vi "Set Tx UDP Properties.vi"(8 "error in":errorcluster, 10 "session_tx_generic":cluster{"portId":u32, "VL":u32}, 11 "custom device ref in":T1 format="%.0x") -> (0 "error out":errorcluster, 3 "custom device ref out":T1 format="%.0x")   [LabVIEW 2020, in "AIM ARINC 664 Scripting.lvlib"]
uses:
  <vilib>/NI VeriStand/Custom Device API/Custom Device Item Ref.ctl
  Constants.vi
  <vilib>/NI VeriStand/Custom Device API/Set Item Property (U32).vi
  AIM ARINC 664 Scripting.lvlib
  <vilib>/NI VeriStand/Custom Device API/Custom Device API.lvlib
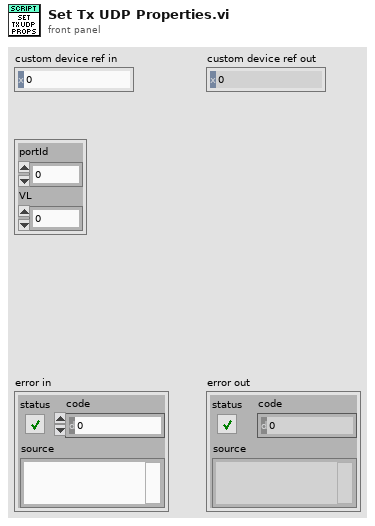
[diagram p1: front panel]
types:
  T1 = typedef "Custom Device API.lvlib/Custom Device Item Ref.ctl" = u64
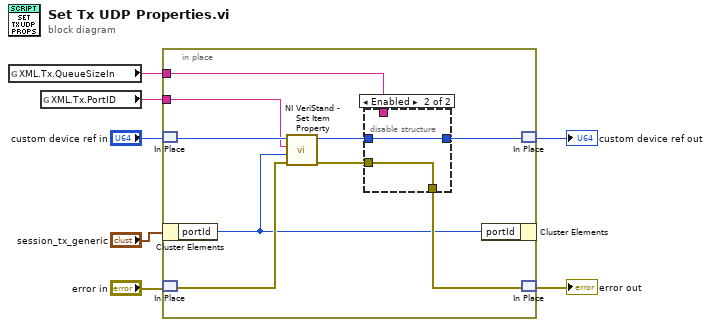
[diagram p0: block diagram]
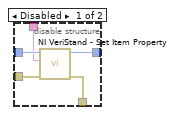
[diagram p2: hidden frame]
diagram:
  n1 = global read "Constants.vi" "XML.Tx.QueueSizeIn"() -> (w3:string)
  n2 = global read "Constants.vi" "XML.Tx.PortID"() -> (w2:string)
  n3 = in-place {
    in-place-border: w3 -> [w9]
    in-place-border: w2 -> [w8]
    n4 = in-place-match #1("custom device ref in") -> (w12:T1)
    n5 = in-place-cluster #2("session_tx_generic") -> ("portId"=w14:u32)
    n6 = in-place-match #3("error in") -> (w16:errorcluster)
    n7 = call-poly <vilib>:"NI VeriStand - Set Item Property.vi"("error in (no error)"=w16, "Value"=w14, "Property Name"=w8, "Item Ref in"=w12) -> ("error out"=w13:errorcluster, "Item Ref out"=w11:T1)  [unwired: 5 in, 1 out]
    n8 = disable-structure shown="Enabled" {
      disable-tunnel: [w21 w23] -> w15
      disable-tunnel: w13 -> [w20 w23]
      disable-tunnel: w11 -> [w19 w22]
      disable-tunnel: [w18 w22] -> w10
      disable-tunnel: w9 -> [w17 _]
      frame Disabled {
        n9 = call-poly <vilib>:"NI VeriStand - Set Item Property.vi"("error in (no error)"=w20, "Property Name"=w17, "Item Ref in"=w19) -> ("error out"=w21:errorcluster, "Item Ref out"=w18:T1)  [unwired: 6 in, 1 out]
      }
      frame Enabled {
      }
    }
    n10 = in-place-cluster #2("portId"=w14) -> ()  [unwired: 1 out]
    n11 = in-place-match #1(w10) -> (→"custom device ref out":T1)
    n12 = in-place-match #3(w15) -> (→"error out":errorcluster)
  }
